vi "Conv_Yards_Meters.vi"(10 "Yards":dbl) -> (2 "Meters":dbl)   [LabVIEW 2019, in "Trajectory_Library.lvlib"]
doc: "Convert Yards to Meters"
uses:
  Trajectory_Library.lvlib
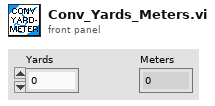
[diagram p1: front panel]
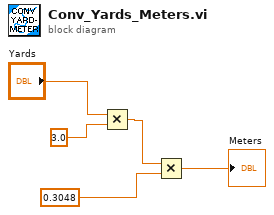
[diagram p0: block diagram]
diagram:
  n1 = Multiply(x="Yards", y=3.0) -> (x*y=w3:dbl)
  n2 = Multiply(x=w3, y=0.3048) -> (x*y=→"Meters":dbl)
